vi "SpectraPro-Control.vi"() -> ()   [LabVIEW 2014]
doc: "Andre Romero - 2016\nandretec@ifsc.usp.br\nIFSC - USP"
panel:
  out "status":bool
  in  "Select grating":u16(ring) items=["Grating 1", "Grating 2"]
  in  "Change":bool
  in  "VISA resource name":refnum<visa-resource-name>="COM12"
  in  "GO TO":bool
  out "return":string="500.00 <GOTO>  ok\r\n"
  in  "Wavelength":dbl=550.0 format="%_5p"
  in  "stop":bool
  # "1 -> 600 - 2400 nm\n2 -> 250 - 800 nm"
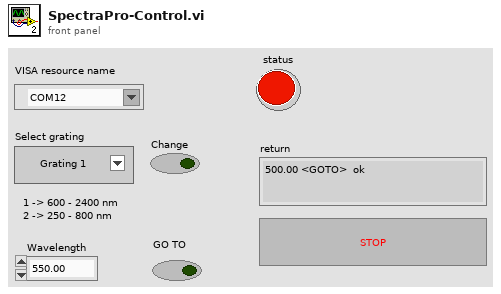
[diagram p1: front panel]
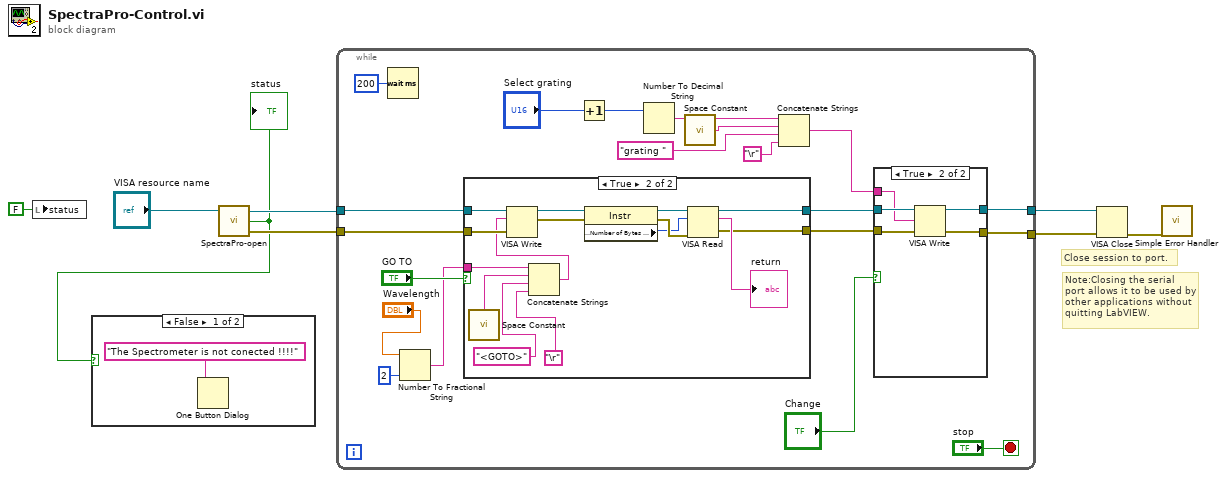
[diagram p0: block diagram]
diagram:
  # "Note:Closing the serial port allows it to be used by other applications without\nquitting LabVIEW."
  # "Close session to port."
  n1 = local write "status"(FALSE ("status")) -> ()
  n2 = call "SpectraPro-open.vi"("VISA resource name"="VISA resource name") -> ("error out"=w4:errorcluster, "status"=w2:bool, "VISA resource name out"=w5:refnum<visa-resource-name>)  [unwired: 2 in]
  "status" <- w2
  n3 = case shown="False" w2 {
    frame False {
      n4 = One Button Dialog(message="The Spectrometer is not conected !!!!") -> ()  [unwired: 1 in, 1 out]
    }
    frame True {
    }
  }
  n5 = while {
    tunnel: w5 -> [w25]
    tunnel: w4 -> [w24]
    tunnel: [w19] -> w7
    tunnel: [w18] -> w6
    stop <- "stop" stop-if-true
    n6 = Wait (ms)(milliseconds to wait=u32 200) -> ()  [unwired: 1 out]
    n7 = Number To Fractional String(number="Wavelength", precision (6)=i16 2) -> (F-format string=w26:string)  [unwired: 2 in]
    n8 = case shown="True" "GO TO" {
      tunnel: w26 -> [_ w51]
      tunnel: w25 -> [w38 w53]
      tunnel: w24 -> [w37 w52]
      tunnel: [w38 w41] -> w21
      tunnel: [w37 w39] -> w20
      frame False {
      }
      frame True {
        n9 = call <vilib>:"Space Constant.vi"() -> ("String"=w50:string)
        n10 = Concatenate Strings(w51, w50, "<GOTO>", "\r") -> (w47:string)
        n11 = VISA Write(VISA resource name=w53, write buffer=w47, error in (no error)=w52) -> (VISA resource name out=w42:refnum<visa-resource-name>, error out=w40:errorcluster)  [unwired: 1 out]
        n12 = property class="Instr"(reference=w42, error in=w40) -> (reference out=w46:refnum<visa-resource-name>, error out=w45:errorcluster, "Serial Settings:Number of Bytes at Serial Port"=w44:u32)
        n13 = VISA Read(VISA resource name=w46, byte count=w44, error in (no error)=w45) -> (VISA resource name out=w41:refnum<visa-resource-name>, read buffer=→"return":string, error out=w39:errorcluster)  [unwired: 1 out]
      }
    }
    n14 = Increment(x="Select grating") -> (x+1=w10:u16)
    n15 = Number To Decimal String(number=w10) -> (decimal integer string=w16:string)  [unwired: 1 in]
    n16 = call <vilib>:"Space Constant.vi"() -> ("String"=w15:string)
    n17 = Concatenate Strings(w16, w15, "grating " ("string"), "\r") -> (w12:string)
    n18 = case shown="True" "Change" {
      tunnel: w21 -> [w31 w36]
      tunnel: w20 -> [w30 w35]
      tunnel: [w31 w34] -> w19
      tunnel: [w30 w33] -> w18
      tunnel: w12 -> [_ w32]
      frame False {
      }
      frame True {
        n19 = VISA Write(VISA resource name=w36, write buffer=w32, error in (no error)=w35) -> (VISA resource name out=w34:refnum<visa-resource-name>, error out=w33:errorcluster)  [unwired: 1 out]
      }
    }
  }
  n20 = VISA Close(VISA resource name=w7, error in (no error)=w6) -> (error out=w8:errorcluster)
  n21 = call <vilib>:"Simple Error Handler.vi"("error in (no error)"=w8) -> ()  [unwired: 4 in, 5 out]
